vi "addI64Element.vi"(7 "Name":string, 8 "error in (no error)":errorcluster, 9 "Value":i64, 10 "Replace? (false)":bool, 11 "tBSONDocument in":refnum<class "tBSONDocument.lvclass">) -> (0 "error out":errorcluster, 3 "tBSONDocument out":refnum<class "tBSONDocument.lvclass">)   [LabVIEW 2013, in "BSON.lvlib" / "tBSONDocument.lvclass"]
doc: "Adds an I64 to a BSON document."
uses:
  tBSONDocument.lvclass
  BSONElements/tBSON_I64/tBSON_I64.lvclass
  tBSONElement/tBSONElement.lvclass
  tBSONElement/setName.vi
  BSONElements/tBSON_I64/setValue.vi
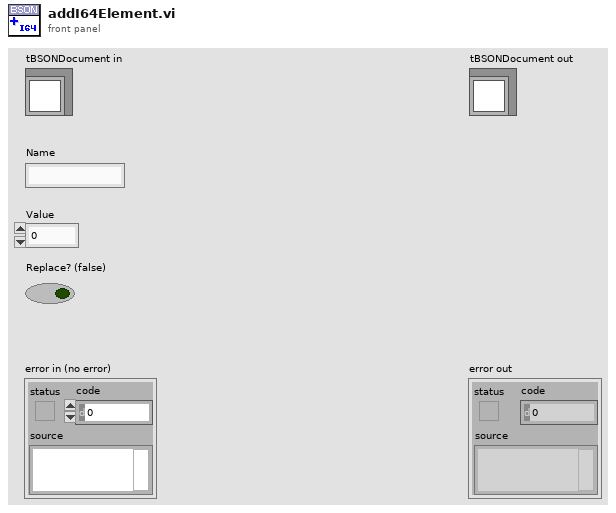
[diagram p1: front panel]
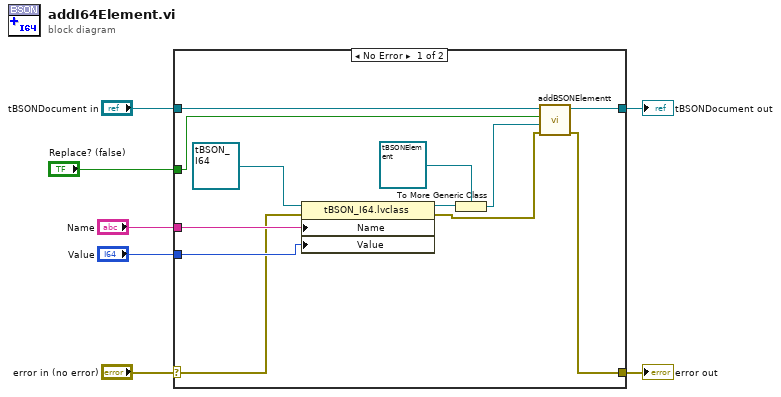
[diagram p0: block diagram]
diagram:
  n1 = case shown="No Error" "error in (no error)" {
    selector: "error in (no error)" -> [w16 w21]
    tunnel: [w10 w21] -> w6
    tunnel: [w9 w20] -> w4
    tunnel: "tBSONDocument in" -> [w13 w20]
    tunnel: "Value" -> [w17 _]
    tunnel: "Name" -> [w18 _]
    tunnel: "Replace? (false)" -> [w8 _]
    frame No Error {
      n2 = property class="tBSON_I64.lvclass"(reference=refnum<class "tBSON_I64.lvclass"> refnum ("BSON.lvlib:tBSON_I64.lvclass"), error in=w16, "Name"=w18, "Value"=w17) -> (reference out=w15:refnum<class "tBSON_I64.lvclass">, error out=w11:errorcluster)
      n3 = To More Generic Class(target class=refnum<class "tBSONElement.lvclass"> refnum ("BSON.lvlib:tBSONElement.lvclass"), reference=w15) -> (generic class reference=w12:refnum<class "tBSONElement.lvclass">)
      n4 = call "addBSONElementt.vi"("error in (no error)"=w11, "Element"=w12, "Replace? (false)"=w8, "tBSONDocument in"=w13) -> ("error out"=w10:errorcluster, "tBSONDocument out"=w9:refnum<class "tBSONDocument.lvclass">)  [unwired: 6 in]
    }
    frame Error {
    }
  }
  "error out" <- w6
  "tBSONDocument out" <- w4
